vi "Get_CCD_temperature_status.vi"(8 "error in":errorcluster, 11 "camera handle in":u64) -> (0 "error out":errorcluster, 1 "PicamSensorTemperatureStatus":T1=1 items=["Unlocked"=1, "Locked"=2, "Faulted"=3], 3 "camera handle out":u64)   [LabVIEW 2014, in "PICam.lvlib"]
doc: "Reads the CCD temperature in Celsius units.\nYou need to call the \"Refresh_parameters_from_camera.vi\" before reading the actual temperature, to receive the updated value from the cam to the local memory.\n\nPicamSensorTemperatureStatus_Unlocked: The temperature has not stabilized at the set\npoint.\nPicamSensorTemperatureStatus_Locked: The temperature has stabilized at the set\npoint."
uses:
  PICam.lvlib
  Ctrls/PicamSensorTemperatureStatus.ctl
  Picam32.dll
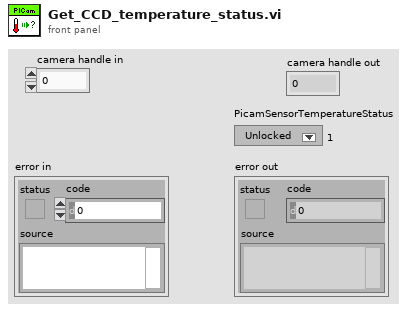
[diagram p1: front panel]
types:
  T1 = typedef "PICam.lvlib/PicamSensorTemperatureStatus.ctl" = u32
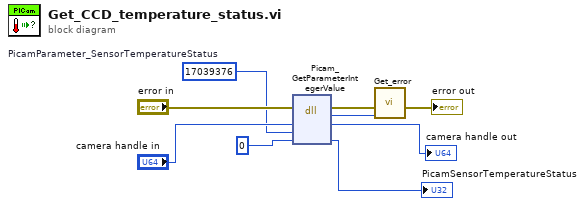
[diagram p0: block diagram]
diagram:
  w5 = u32 17039376  # PicamParameter_SensorTemperatureStatus
  n1 = dll-call lib="Picam32.dll" fn="Picam_GetParameterIntegerValue"(error in="error in", "camera"="camera handle in", "PicamParameter"=w5, "temperature_status"=u32 0) -> (error out=w9:errorcluster, "return type"=w8:i32, "camera"=→"camera handle out":u64, "temperature_status"=→"PicamSensorTemperatureStatus":u32)  [unwired: 3 in, 1 out]
  n2 = call "Get_error.vi"("PICam_Error"=w8, "error in (no error)"=w9) -> ("error out"=→"error out":errorcluster)  [unwired: 9 in]
